vi "EX 4-1 Analog Read Pin.vi"() -> ()   [LabVIEW 2011, in "LabVIEW Interface for Arduino.lvlib"]
doc: "An example that reads a user selectable analog input pin on the Arduino."
uses:
  <vilib>/LabVIEW Interface for Arduino/LabVIEW Interface for Arduino.lvlib
  <vilib>/LabVIEW Interface for Arduino/Type Defs/Analog Pin.ctl
  <vilib>/LabVIEW Interface for Arduino/Type Defs/Board Type.ctl
panel:
  in  "Analog Pin":T1
  in  "Stop":bool
  out "Voltage":dbl(knob) scale=0.0..5.0
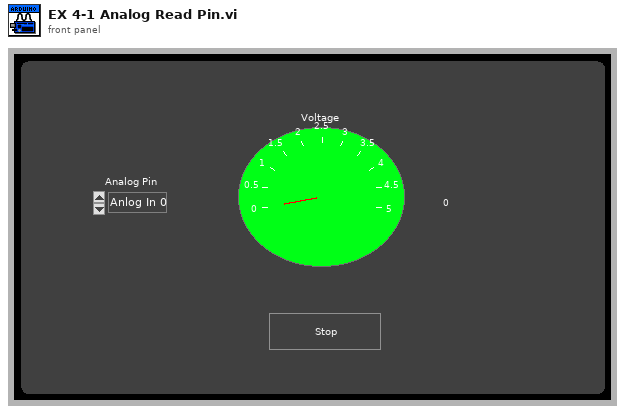
[diagram p1: front panel]
types:
  T1 = typedef "LabVIEW Interface for Arduino.lvlib/Analog Pin.ctl" = enum8{"Anlog In 0", "Anlog In 1", "Anlog In 2", "Anlog In 3", "Anlog In 4", "Anlog In 5"}
  T2 = typedef "LabVIEW Interface for Arduino.lvlib/Board Type.ctl" = enum16{"Uno", "Dimuelanove w/Atmega 328", "Mega 2560"}
  T3 = typedef "LabVIEW Interface for Arduino.lvlib/Arduino Resource.ctl" = cluster{"VISA resource":refnum<visa-resource-name>, "Board Type":T2, "Connection Type":enum8{"USB / Serial"}, "Bytes Per Packet (15)":u8}
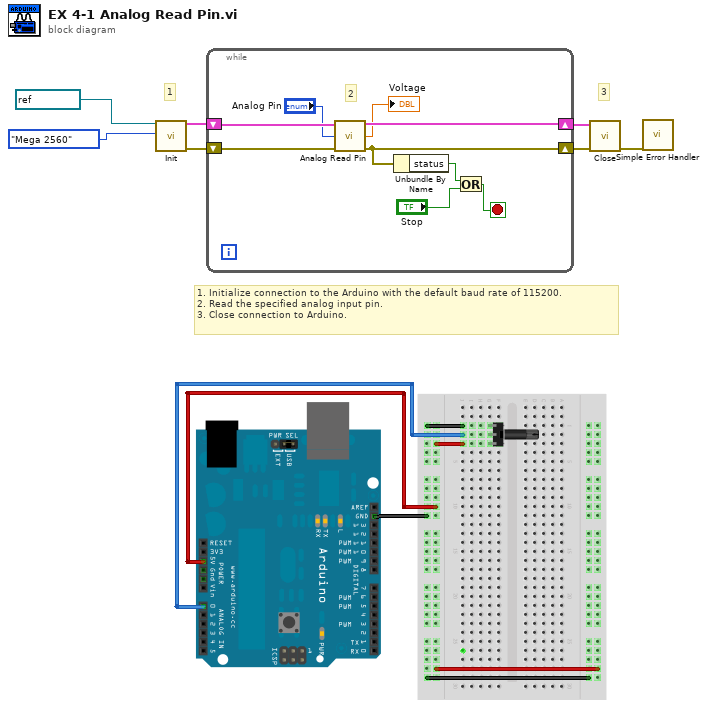
[diagram p0: block diagram]
diagram:
  # "1. Initialize connection to the Arduino with the default baud rate of 115200.\n2. Read the specified analog input pin.\n3. Close connection to Arduino."
  # "3"
  # "1"
  n1 = call <vilib>:"Init.vi"("VISA resource"=refnum<visa-resource-name> "COM9", "Board Type (Uno)"=Board_Type."Mega 2560") -> ("Arduino Resource"=w7:T3, "error out"=w4:errorcluster)  [unwired: 16 in]
  n2 = while {
    shift-right: [w16] -> w6
    shift-left: w7 -> [w10]
    shift-right: [w14] -> w5
    shift-left: w4 -> [w9]
    stop <- w13 stop-if-true
    # "2"
    n3 = call <vilib>:"Analog Read Pin.vi"("Arduino Resource"=w10, "Analog Input Pin (0)"="Analog Pin", "error in"=w9) -> ("Arduino Resource"=w16:T3, "Voltage"=→"Voltage":dbl, "error out"=w14:errorcluster)  [unwired: 10 in]
    n4 = Unbundle By Name(w14) -> ("status"=w12:bool)
    n5 = Or(x=w12, y="Stop") -> (x .or. y?=w13:bool)
  }
  n6 = call <vilib>:"Close.vi"("Arduino Resource"=w6, "error in"=w5) -> ("error out"=w3:errorcluster)  [unwired: 13 in]
  n7 = call <vilib>:"Simple Error Handler.vi"("error in (no error)"=w3) -> ()  [unwired: 4 in, 5 out]
